vi "Modulation_Freqs_Orders.vi"(7 "Multiple_Frequency":i32=3, 11 "char freqs":T2) -> (1 "char orders out":T1[][](array[typedef]), 3 "char freqs out":T1[][](array[typedef]))   [LabVIEW 2021]
uses:
  Typedefs/Detected peaks.ctl
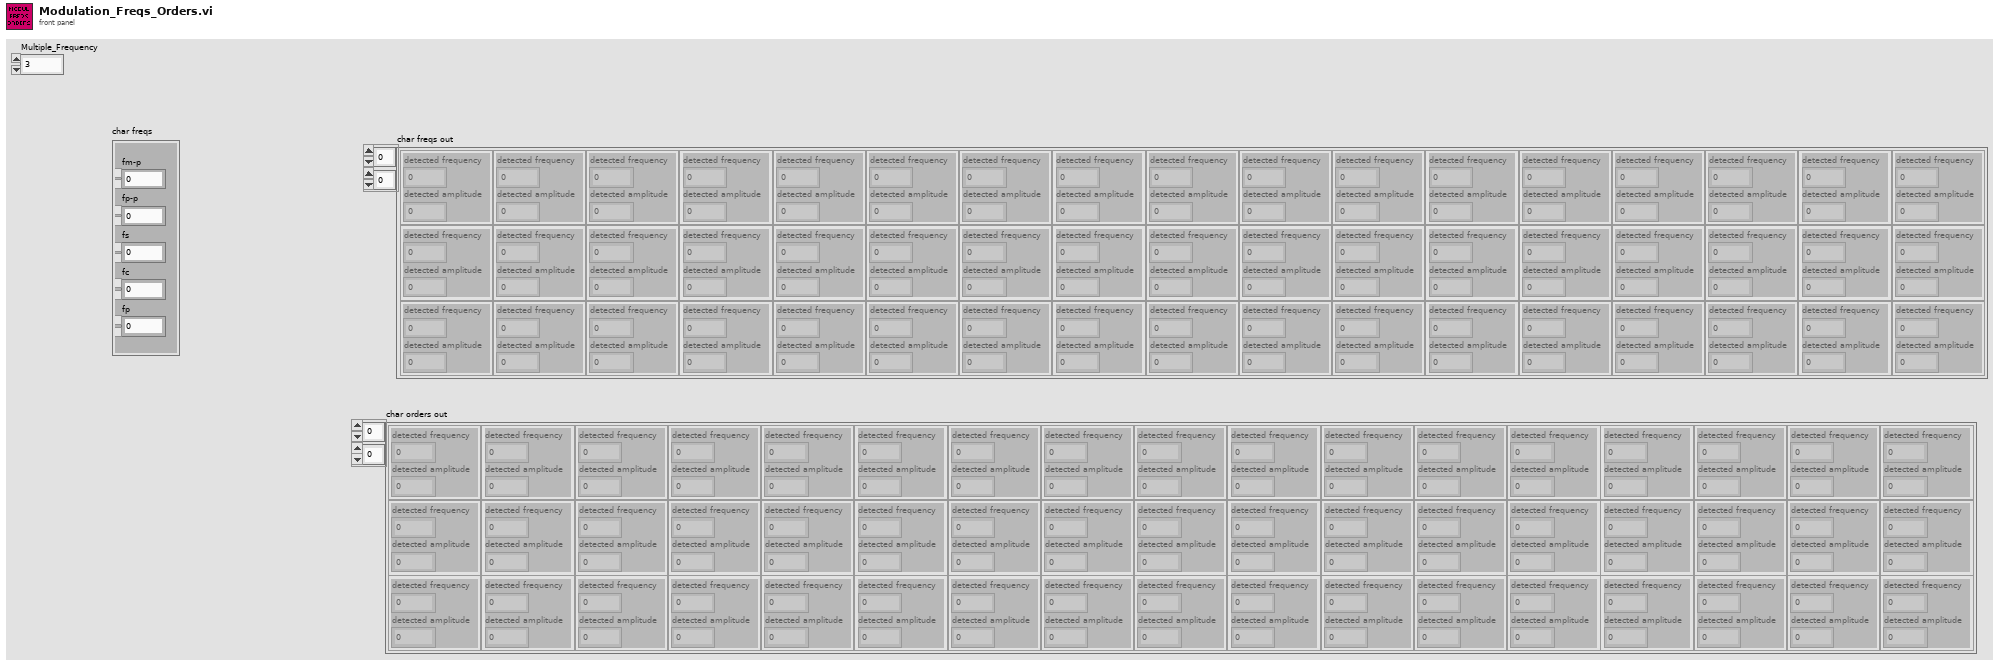
[diagram p1: front panel]
types:
  T1 = typedef "Detected peaks.ctl" = cluster{"detected frequency":dbl, "detected amplitude":dbl}
  T2 = cluster{"fm-p":dbl, "fp-p":dbl, "fs":dbl, "fc":dbl, "fp":dbl}
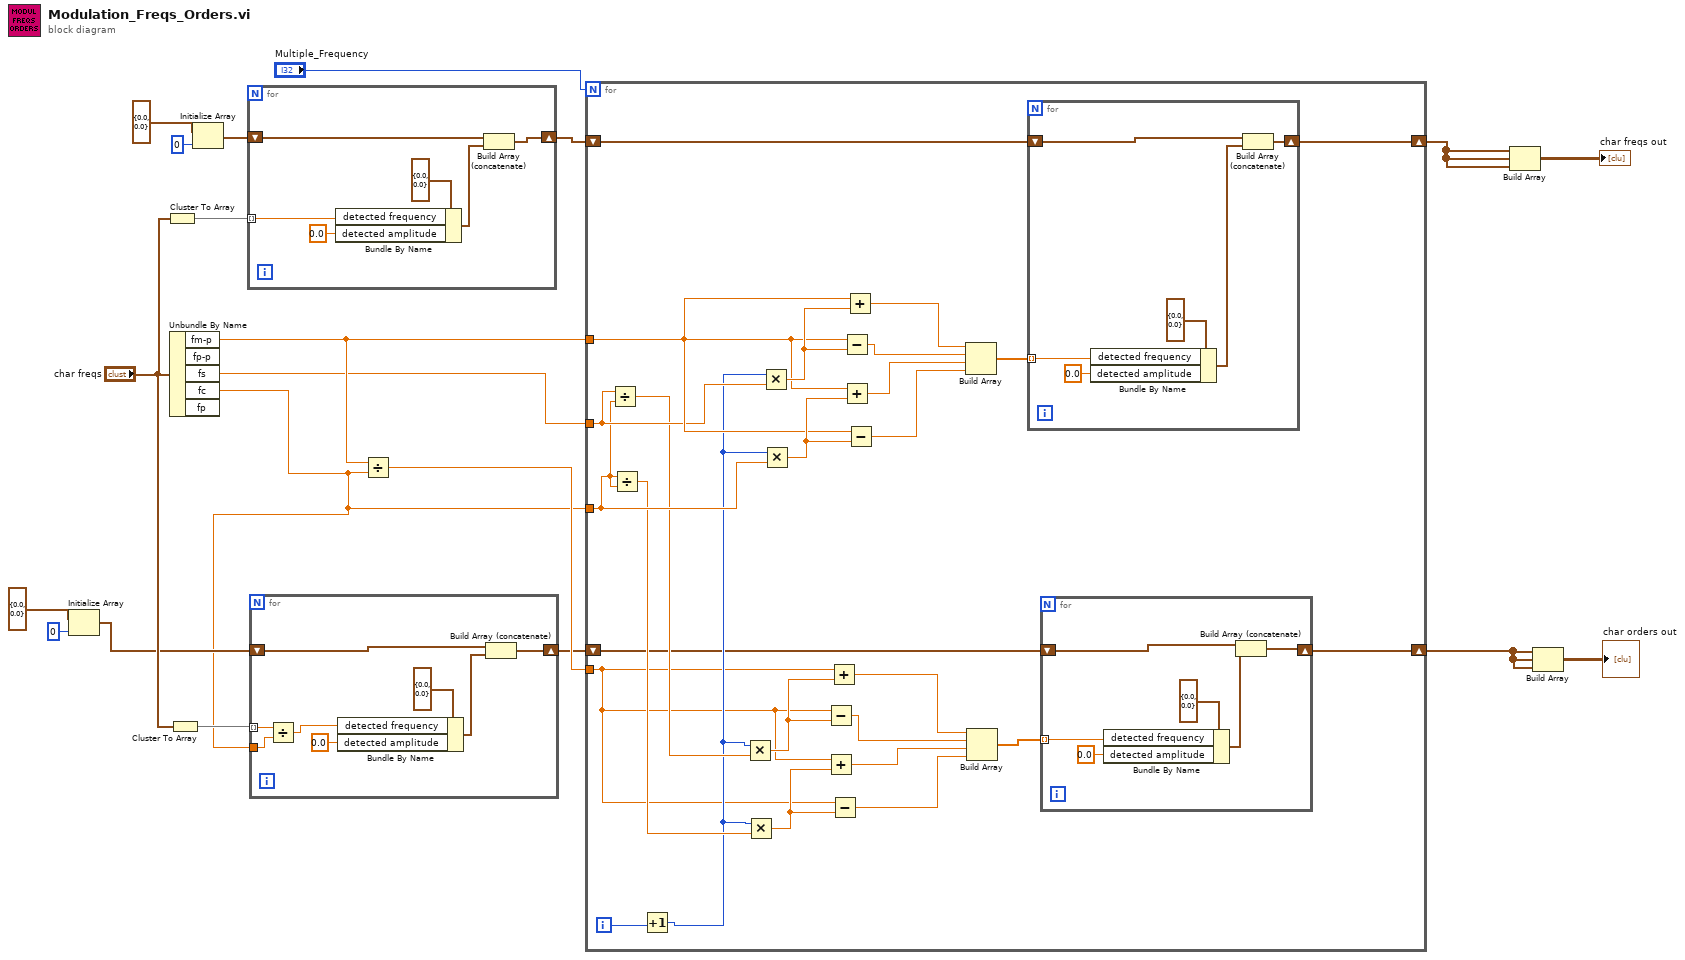
[diagram p0: block diagram]
diagram:
  n1 = Initialize Array(T1 {"detected frequency"=0.0, "detected amplitude"=0.0}, 0 ("dimension size")) -> (w6:T1[])
  n2 = Cluster To Array(cluster="char freqs") -> (array=w17:dbl[])
  n3 = Unbundle By Name("char freqs") -> ("fm-p"=w19:dbl, "fs"=w18:dbl, "fc"=w4:dbl)  [unwired: 2 out]
  n4 = Cluster To Array(cluster="char freqs") -> (array=w9:dbl[])
  n5 = Initialize Array(T1 {"detected frequency"=0.0, "detected amplitude"=0.0}, 0 ("dimension size")) -> (w15:T1[])
  n6 = for {
    tunnel: w17 -> [w24] mode=indexing
    shift-right: [w21] -> w14
    shift-left: w15 -> [w23]
    n7 = Bundle By Name(cluster=T1 {"detected frequency"=0.0, "detected amplitude"=0.0}, "detected frequency"=w24, "detected amplitude"=0.0) -> (w22:T1)
    n8 = Build Array (concatenate)(w23, w22) -> (w21:T1[])
  }
  n9 = for {
    tunnel: w9 -> [w29] mode=indexing
    shift-right: [w30] -> w5
    shift-left: w6 -> [w32]
    tunnel: w4 -> [w28]
    n10 = Divide(x=w29, y=w28) -> (x/y=w27:dbl)
    n11 = Bundle By Name(cluster=T1 {"detected frequency"=0.0, "detected amplitude"=0.0}, "detected frequency"=w27, "detected amplitude"=0.0) -> (w31:T1)
    n12 = Build Array (concatenate)(w32, w31) -> (w30:T1[])
  }
  n13 = Divide(x=w19, y=w4) -> (x/y=w20:dbl)
  n14 = for {
    N: "Multiple_Frequency" -> [_]
    tunnel: w19 -> [w54]
    tunnel: w18 -> [w53]
    tunnel: w4 -> [w52]
    tunnel: w20 -> [w41]
    shift-right: [w38] -> w12
    shift-left: w14 -> [w39]
    shift-right: [w35] -> w3
    shift-left: w5 -> [w36]
    i -> [w43]
    n15 = Divide(x=w53, y=w52) -> (x/y=w48:dbl)
    n16 = Divide(x=w52, y=w52) -> (x/y=w49:dbl)
    n17 = Increment(x=w43) -> (x+1=w42:i32)
    n18 = Multiply(x=w42, y=w48) -> (x*y=w50:dbl)
    n19 = Multiply(x=w42, y=w49) -> (x*y=w51:dbl)
    n20 = Multiply(x=w42, y=w53) -> (x*y=w60:dbl)
    n21 = Multiply(x=w42, y=w52) -> (x*y=w59:dbl)
    n22 = Subtract(x=w41, y=w50) -> (x-y=w46:dbl)
    n23 = Add(x=w41, y=w51) -> (x+y=w45:dbl)
    n24 = Add(x=w41, y=w50) -> (x+y=w47:dbl)
    n25 = Subtract(x=w41, y=w51) -> (x-y=w44:dbl)
    n26 = Subtract(x=w54, y=w60) -> (x-y=w57:dbl)
    n27 = Add(x=w54, y=w59) -> (x+y=w56:dbl)
    n28 = Add(x=w54, y=w60) -> (x+y=w58:dbl)
    n29 = Subtract(x=w54, y=w59) -> (x-y=w55:dbl)
    n30 = Build Array(w58, w57, w56, w55) -> (w40:dbl[])
    n31 = Build Array(w47, w46, w45, w44) -> (w37:dbl[])
    n32 = for {
      tunnel: w40 -> [w70] mode=indexing
      shift-right: [w67] -> w38
      shift-left: w39 -> [w69]
      n33 = Bundle By Name(cluster=T1 {"detected frequency"=0.0, "detected amplitude"=0.0}, "detected frequency"=w70, "detected amplitude"=0.0) -> (w68:T1)
      n34 = Build Array (concatenate)(w69, w68) -> (w67:T1[])
    }
    n35 = for {
      tunnel: w37 -> [w64] mode=indexing
      shift-right: [w61] -> w35
      shift-left: w36 -> [w63]
      n36 = Bundle By Name(cluster=T1 {"detected frequency"=0.0, "detected amplitude"=0.0}, "detected frequency"=w64, "detected amplitude"=0.0) -> (w62:T1)
      n37 = Build Array (concatenate)(w63, w62) -> (w61:T1[])
    }
  }
  n38 = Build Array(w12, w12, w12) -> (→"char freqs out":T1[][])
  n39 = Build Array(w3, w3, w3) -> (→"char orders out":T1[][])
